vi "save_summed_trace.vi"(0 "start path":path=path "", 2 "Channel":u16(ring) items=["C1", "C2"], 7 "Complete Data cluster":T1, 11 "error in (no error)":errorcluster, 13 "Variables Cluster":T2) -> (15 "error out":errorcluster)   [LabVIEW 2023]
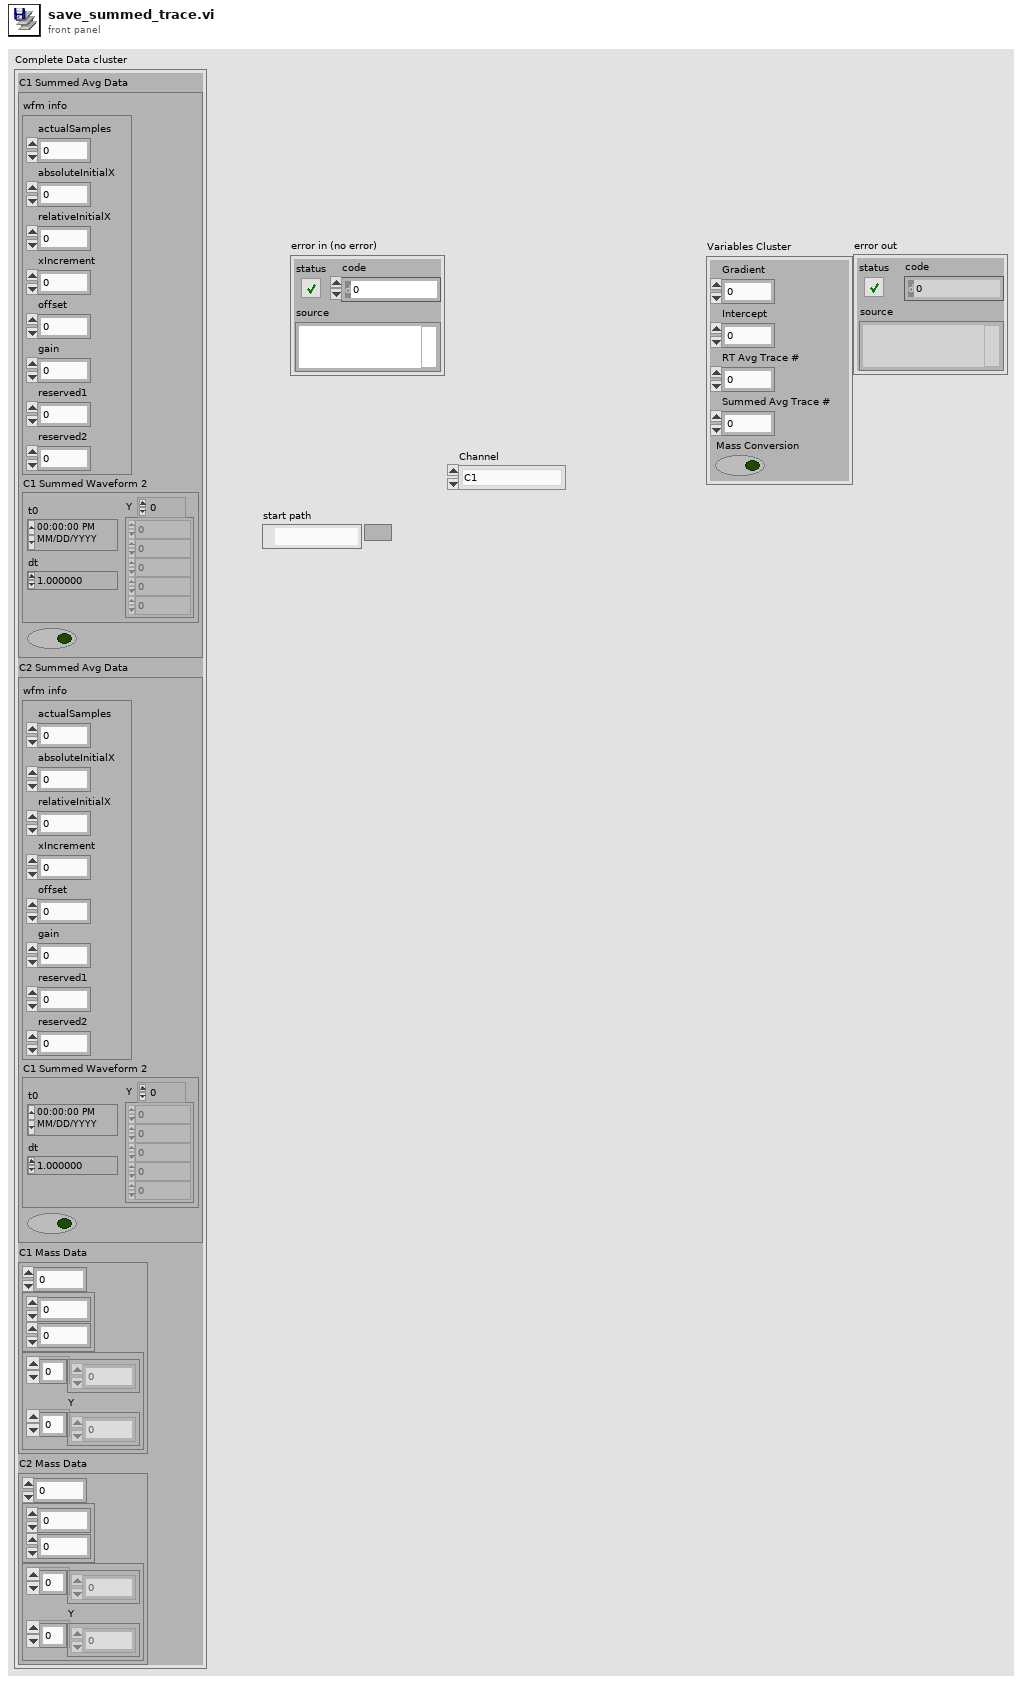
[diagram p1: front panel]
types:
  T1 = cluster{"C1 Summed Avg Data":cluster{"wfm info":cluster{"actualSamples":i32, "absoluteInitialX":dbl, "relativeInitialX":dbl, "xIncrement":dbl, "offset":dbl, "gain":dbl, "reserved1":dbl, "reserved2":dbl}, "C1 Summed Waveform 2":waveform(dbl), bool}, "C2 Summed Avg Data":cluster{"wfm info":cluster{"actualSamples":i32, "absoluteInitialX":dbl, "relativeInitialX":dbl, "xIncrement":dbl, "offset":dbl, "gain":dbl, "reserved1":dbl, "reserved2":dbl}, "C1 Summed Waveform 2":waveform(dbl), bool}, "C1 Mass Data":cluster{dbl, cluster{dbl, dbl}, cluster{dbl[], "Y":dbl[]}}, "C2 Mass Data":cluster{dbl, cluster{dbl, dbl}, cluster{dbl[], "Y":dbl[]}}}
  T2 = cluster{"Gradient":dbl, "Intercept":dbl, "RT Avg Trace #":i32, "Summed Avg Trace #":i32, "Mass Conversion":bool}
  T3 = cluster{"wfm info":cluster{"actualSamples":i32, "absoluteInitialX":dbl, "relativeInitialX":dbl, "xIncrement":dbl, "offset":dbl, "gain":dbl, "reserved1":dbl, "reserved2":dbl}, "C1 Summed Waveform 2":waveform(dbl), bool}
  T4 = cluster{dbl, cluster{dbl, dbl}, cluster{dbl[], "Y":dbl[]}}
  T5 = cluster{"actualSamples":i32, "absoluteInitialX":dbl, "relativeInitialX":dbl, "xIncrement":dbl, "offset":dbl, "gain":dbl, "reserved1":dbl, "reserved2":dbl}
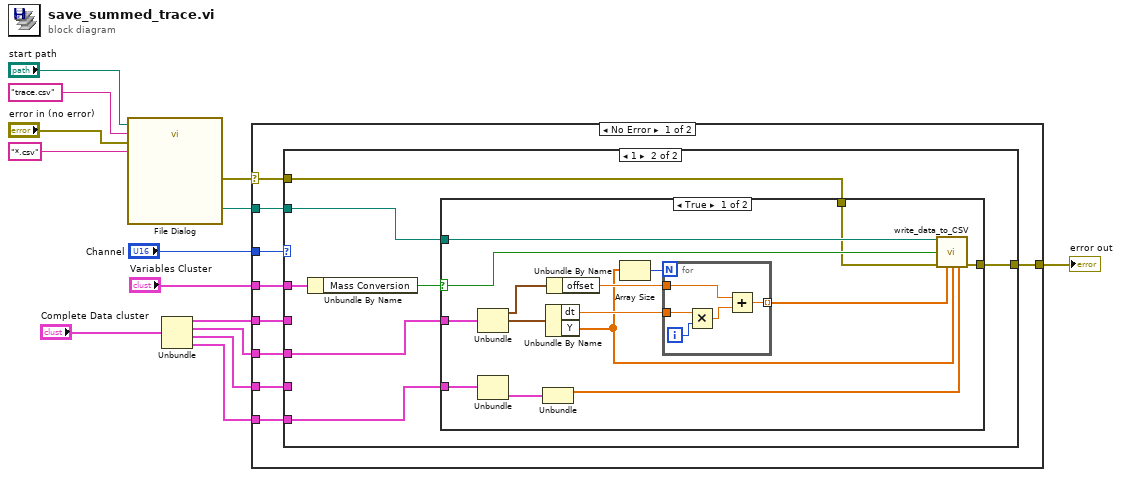
[diagram p0: block diagram]
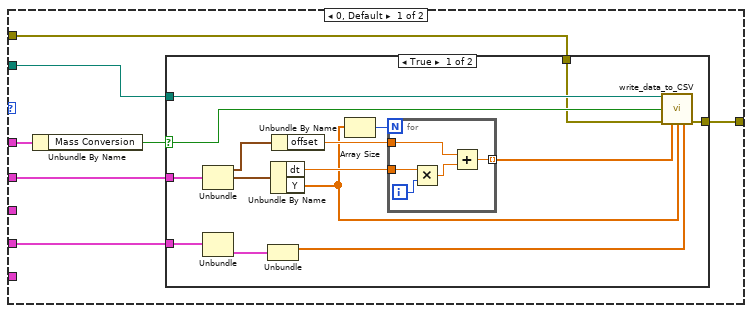
[diagram p2: hidden frame]
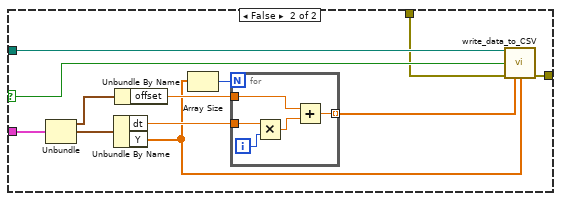
[diagram p3: hidden frame]
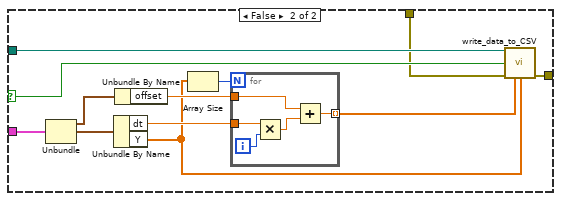
[diagram p4: hidden frame]
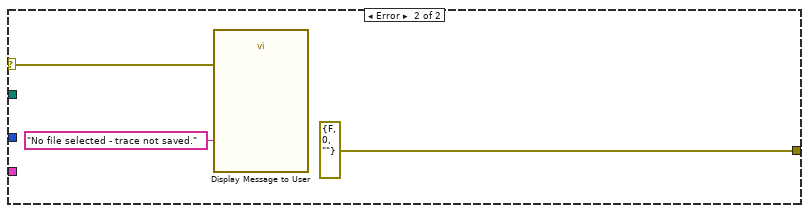
[diagram p5: hidden frame]
diagram:
  n1 = call "File Dialog"("start path"="start path", "default name"="trace.csv", "error in"="error in (no error)", "pattern (all files)"="*.csv") -> ("selected path"=w14:path, "error out"=w10:errorcluster)  [unwired: 8 in, 2 out]
  n2 = Unbundle("Complete Data cluster") -> ("C1 Summed Avg Data"=w4:T3, "C2 Summed Avg Data"=w3:T3, "C1 Mass Data"=w2:T4, "C2 Mass Data"=w1:T4)
  n3 = case shown="No Error" w10 {
    selector: w10 -> [w16 w114]
    tunnel: w14 -> [w23 _]
    tunnel: "Channel" -> [w22 _]
    tunnel: w4 -> [w21 _]
    tunnel: w3 -> [w20 _]
    tunnel: w2 -> [w19 _]
    tunnel: w1 -> [w18 _]
    tunnel: "Variables Cluster" -> [w17 _]
    tunnel: [w15 errorcluster {"status"=FALSE, "code"=0, "source"=""} ("error out")] -> w6
    frame No Error {
      n4 = case shown="1" w22 {
        tunnel: w23 -> [w26 w72]
        tunnel: w21 -> [w28 _]
        tunnel: w20 -> [_ w69]
        tunnel: w19 -> [w27 _]
        tunnel: w18 -> [_ w68]
        tunnel: w17 -> [w30 w74]
        tunnel: w16 -> [w25 w71]
        tunnel: [w24 w70] -> w15
        frame 0, Default {
          n5 = Unbundle By Name(w30) -> ("Mass Conversion"=w29:bool)
          n6 = case shown="True" w29 {
            selector: w29 -> [w38 w55]
            tunnel: w28 -> [w45 w62]
            tunnel: w27 -> [w35 _]
            tunnel: w26 -> [w39 w56]
            tunnel: [w32 w52] -> w24
            tunnel: w25 -> [w31 w51]
            frame True {
              n7 = Unbundle(w45) -> ("wfm info"=w42:T5, "C1 Summed Waveform 2"=w44:waveform(dbl))  [unwired: 1 out]
              n8 = Unbundle(w35) -> (w34:cluster{dbl[], "Y":dbl[]})  [unwired: 2 out]
              n9 = Unbundle(w34) -> (w33:dbl[])  [unwired: 1 out]
              n10 = Unbundle By Name(w44) -> ("dt"=w43:dbl, "Y"=w36:dbl[])
              n11 = Unbundle By Name(w42) -> ("offset"=w41:dbl)
              n12 = Array Size(array=w36) -> (size(s)=w40:i32)
              n13 = for {
                N: w40 -> [_]
                tunnel: w43 -> [w50]
                tunnel: w41 -> [w47]
                tunnel: [w46] -> w37 mode=indexing
                i -> [w49]
                n14 = Multiply(x=w50, y=w49) -> (x*y=w48:dbl)
                n15 = Add(x=w47, y=w48) -> (x+y=w46:dbl)
              }
              n16 = call "write_data_to_CSV.vi"("file path (dialog if empty)"=w39, "Show mass domain?"=w38, "error in (no error)"=w31, "Time data"=w37, "Intensity data"=w36, "Mass data"=w33) -> ("error out"=w32:errorcluster)  [unwired: 9 in]
            }
            frame False {
              n17 = Unbundle(w62) -> ("wfm info"=w59:T5, "C1 Summed Waveform 2"=w61:waveform(dbl))  [unwired: 1 out]
              n18 = Unbundle By Name(w61) -> ("dt"=w60:dbl, "Y"=w53:dbl[])
              n19 = Unbundle By Name(w59) -> ("offset"=w58:dbl)
              n20 = Array Size(array=w53) -> (size(s)=w57:i32)
              n21 = for {
                N: w57 -> [_]
                tunnel: w60 -> [w67]
                tunnel: w58 -> [w64]
                tunnel: [w63] -> w54 mode=indexing
                i -> [w66]
                n22 = Multiply(x=w67, y=w66) -> (x*y=w65:dbl)
                n23 = Add(x=w64, y=w65) -> (x+y=w63:dbl)
              }
              n24 = call "write_data_to_CSV.vi"("file path (dialog if empty)"=w56, "Show mass domain?"=w55, "error in (no error)"=w51, "Time data"=w54, "Intensity data"=w53) -> ("error out"=w52:errorcluster)  [unwired: 10 in]
            }
          }
        }
        frame 1 {
          n25 = Unbundle By Name(w74) -> ("Mass Conversion"=w73:bool)
          n26 = case shown="True" w73 {
            selector: w73 -> [w82 w99]
            tunnel: w69 -> [w89 w106]
            tunnel: w68 -> [w79 _]
            tunnel: w72 -> [w83 w100]
            tunnel: [w76 w96] -> w70
            tunnel: w71 -> [w75 w95]
            frame True {
              n27 = Unbundle(w89) -> ("wfm info"=w86:T5, "C1 Summed Waveform 2"=w88:waveform(dbl))  [unwired: 1 out]
              n28 = Unbundle(w79) -> (w78:cluster{dbl[], "Y":dbl[]})  [unwired: 2 out]
              n29 = Unbundle(w78) -> (w77:dbl[])  [unwired: 1 out]
              n30 = Unbundle By Name(w88) -> ("dt"=w87:dbl, "Y"=w80:dbl[])
              n31 = Unbundle By Name(w86) -> ("offset"=w85:dbl)
              n32 = Array Size(array=w80) -> (size(s)=w84:i32)
              n33 = for {
                N: w84 -> [_]
                tunnel: w87 -> [w94]
                tunnel: w85 -> [w91]
                tunnel: [w90] -> w81 mode=indexing
                i -> [w93]
                n34 = Multiply(x=w94, y=w93) -> (x*y=w92:dbl)
                n35 = Add(x=w91, y=w92) -> (x+y=w90:dbl)
              }
              n36 = call "write_data_to_CSV.vi"("file path (dialog if empty)"=w83, "Show mass domain?"=w82, "error in (no error)"=w75, "Time data"=w81, "Intensity data"=w80, "Mass data"=w77) -> ("error out"=w76:errorcluster)  [unwired: 9 in]
            }
            frame False {
              n37 = Unbundle(w106) -> ("wfm info"=w103:T5, "C1 Summed Waveform 2"=w105:waveform(dbl))  [unwired: 1 out]
              n38 = Unbundle By Name(w105) -> ("dt"=w104:dbl, "Y"=w97:dbl[])
              n39 = Unbundle By Name(w103) -> ("offset"=w102:dbl)
              n40 = Array Size(array=w97) -> (size(s)=w101:i32)
              n41 = for {
                N: w101 -> [_]
                tunnel: w104 -> [w111]
                tunnel: w102 -> [w108]
                tunnel: [w107] -> w98 mode=indexing
                i -> [w110]
                n42 = Multiply(x=w111, y=w110) -> (x*y=w109:dbl)
                n43 = Add(x=w108, y=w109) -> (x+y=w107:dbl)
              }
              n44 = call "write_data_to_CSV.vi"("file path (dialog if empty)"=w100, "Show mass domain?"=w99, "error in (no error)"=w95, "Time data"=w98, "Intensity data"=w97) -> ("error out"=w96:errorcluster)  [unwired: 10 in]
            }
          }
        }
      }
    }
    frame Error {
      n45 = call "Display Message to User"("error in (no error)"=w114, "Message"="No file selected - trace not saved.") -> ()  [unwired: 8 in, 2 out]
    }
  }
  "error out" <- w6
